vi "Excel Duplicate WorkSheet.vi"(7 "Position (F: before, T: after)":bool=TRUE, 8 "error in (no error)":errorcluster, 9 "New Sheet":string, 10 "Source Sheet":string, 11 "report in":refnum<class "NI_report.lvclass">) -> (0 "error out":errorcluster, 2 "Excel._Worksheet New reference out":refnum<k7>, 3 "report out":refnum<class "NI_report.lvclass">)   [LabVIEW 2020, in "varilib.lvlib"]
doc: "Duplicate worksheet in excel file. \"Source sheet\" is copied and named by the name \"New Sheet\". If the name \"New Sheet\" is not set or empty string, the name of the new sheet will be automatically generated by excel, i.e. \"Source sheet (2)\", or in the case last characters of \"Source sheet\" are \"(n)\", \"Source sheet (n+1)\". The position of the new worksheet is before the source sheet, or after."
uses:
  varilib.lvlib
  <vilib>/Utility/NIReport.llb/Excel/NI_Excel.lvclass
  <vilib>/Utility/NIReport.llb/NI_report.lvclass
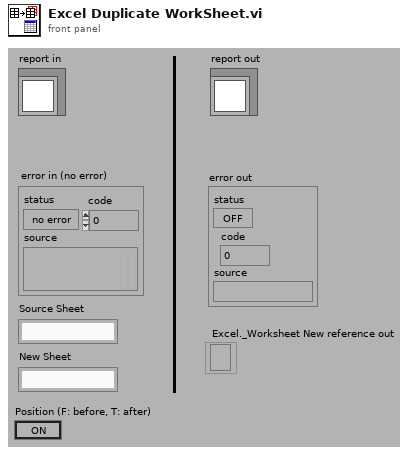
[diagram p1: front panel]
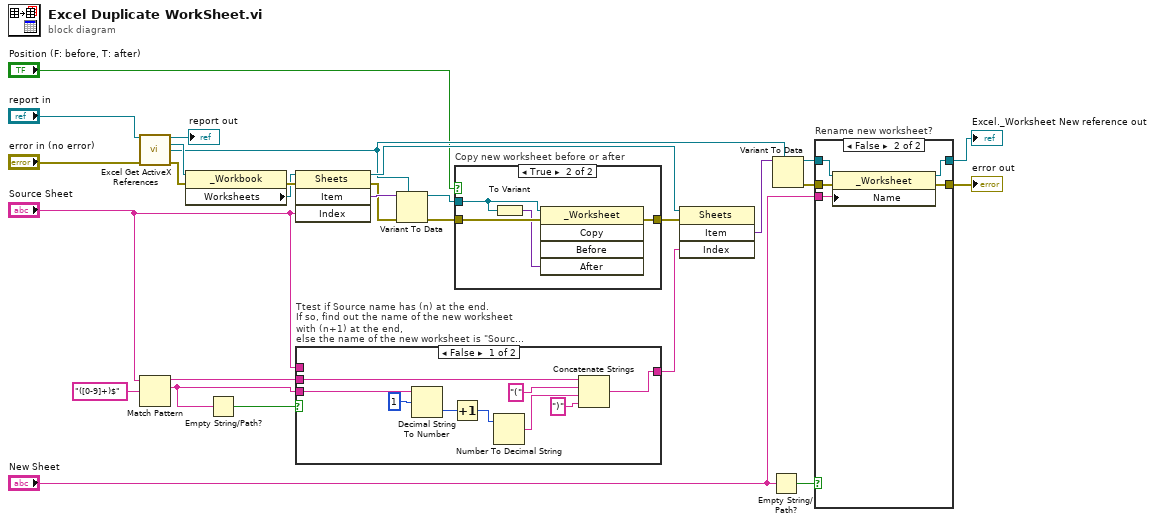
[diagram p0: block diagram]
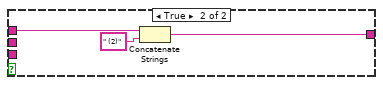
[diagram p2: hidden frame]
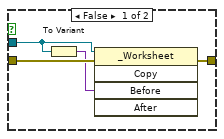
[diagram p4: hidden frame]
diagram:
  n1 = call <vilib>:"Excel Get ActiveX References.vi"("report in"="report in", "error in (no error)"="error in (no error)") -> ("report out"=→"report out":refnum<class "NI_report.lvclass">, "Excel._Workbook"=w10:refnum<k7>, "Excel._Worksheet"=w9:refnum<k7>, "error out"=w13:errorcluster)  [unwired: 7 in, 3 out]
  n2 = Match Pattern(string="Source Sheet", regular expression="([0-9]+)$") -> (before substring=w1:string, match substring=w2:string)  [unwired: 1 in, 2 out]
  n3 = property class="_Workbook"(reference=w10, error in=w13) -> (error out=w25:errorcluster, "Worksheets"=w23:refnum<k7>)  [unwired: 1 out]
  n4 = Empty String/Path?(string/path=w2) -> (empty?=w3:bool)
  n5 = invoke class="Sheets" method="Item"(reference=w23, error in=w25, "Index"="Source Sheet") -> (reference out=w21:refnum<k7>, error out=w27:errorcluster, "Item"=w28:variant)  [unwired: 1 in, 1 out]
  n6 = case "Ttest if Source name has (n) at the end.\nIf so, find out the name of the new worksheet with (n+1) at the end,\nelse the name of the new worksheet is \"Source name (2)\"" shown="False" w3 {
    tunnel: [w29 w39] -> w20
    tunnel: "Source Sheet" -> [_ w38]
    tunnel: w2 -> [w36 _]
    tunnel: w1 -> [w35 _]
    frame False {
      n7 = Decimal String To Number(string=w36, offset=1) -> (number=w34:i32)  [unwired: 1 in, 1 out]
      n8 = Increment(x=w34) -> (x+1=w32:i32)
      n9 = Number To Decimal String(number=w32) -> (decimal integer string=w31:string)  [unwired: 1 in]
      n10 = Concatenate Strings(w35, "(" ("string"), w31, ")" ("string")) -> (w29:string)
    }
    frame True {
      n11 = Concatenate Strings(w38, " (2)") -> (w39:string)
    }
  }
  n12 = Variant To Data(error in=w27, type=w9, Variant=w28) -> (data=w24:refnum<k7>, error out=w26:errorcluster)
  n13 = case "Copy new worksheet before or after" shown="True" "Position (F: before, T: after)" {
    tunnel: w26 -> [w44 w48]
    tunnel: w24 -> [w43 w47]
    tunnel: [w42 w45] -> w22
    frame False {
      n14 = To Variant(anything=w43) -> (Variant=w41:variant)
      n15 = invoke class="_Worksheet" method="Copy"(reference=w43, error in=w44, "Before"=w41) -> (error out=w42:errorcluster)  [unwired: 2 in, 4 out]
    }
    frame True {
      n16 = To Variant(anything=w47) -> (Variant=w46:variant)
      n17 = invoke class="_Worksheet" method="Copy"(reference=w47, error in=w48, "After"=w46) -> (error out=w45:errorcluster)  [unwired: 2 in, 4 out]
    }
  }
  n18 = invoke class="Sheets" method="Item"(reference=w21, error in=w22, "Index"=w20) -> ("Item"=w19:variant)  [unwired: 1 in, 3 out]
  n19 = Empty String/Path?(string/path="New Sheet") -> (empty?=w6:bool)
  n20 = Variant To Data(type=w9, Variant=w19) -> (data=w17:refnum<k7>, error out=w18:errorcluster)  [unwired: 1 in]
  n21 = case "Rename new worksheet?" shown="False" w6 {
    tunnel: w18 -> [w49 w55]
    tunnel: w17 -> [w50 w54]
    tunnel: [w50 w53] -> w16
    tunnel: [w49 w52] -> w15
    tunnel: "New Sheet" -> [_ w51]
    frame True {
    }
    frame False {
      n22 = property class="_Worksheet"(reference=w54, error in=w55, "Name"=w51) -> (reference out=w53:refnum<k7>, error out=w52:errorcluster)
    }
  }
  "error out" <- w15
  "Excel._Worksheet New reference out" <- w16
